vi "xiC - IMAQ - UpdateXiControl.vi"(6 "PRM_Attributes":T1={"Type"=enum."Int32", "Method"=enum."Get / Set", "Desc."="", "PRM"=enum."DEVICE_NAME"}, 8 "error in (no error)":errorcluster, 11 "Attributes In":T5) -> (0 "error out":errorcluster, 3 "Attributes Out":T5)   [LabVIEW 2015]
uses:
  xiCamLib/xiLIB/Typedefs/xiLIB - PRM_Function.ctl
  xiC - IMAQ - Attributes.ctl
  C:/GIT/Cameras3.x/Integrations/Labview/xiLib/xiLIB_32bit/xiLIB/xiCamLib/API/x86/xiApi.NET.dll
  xiLIB_32bit/xiLIB/xiCamLib/API/x86/xiApi.NET.dll
  xiCamLib/xiLIB/Typedefs/xiLIB - PRM_Type.ctl
  xiCamLib/xiLIB/Typedefs/xiLIB - PRM_Attribute.ctl
  xiC - IMAQ - TreeDisplayType.ctl
  xiCamLib/xiCam/PRM/PRM/PRM_v2.ctl
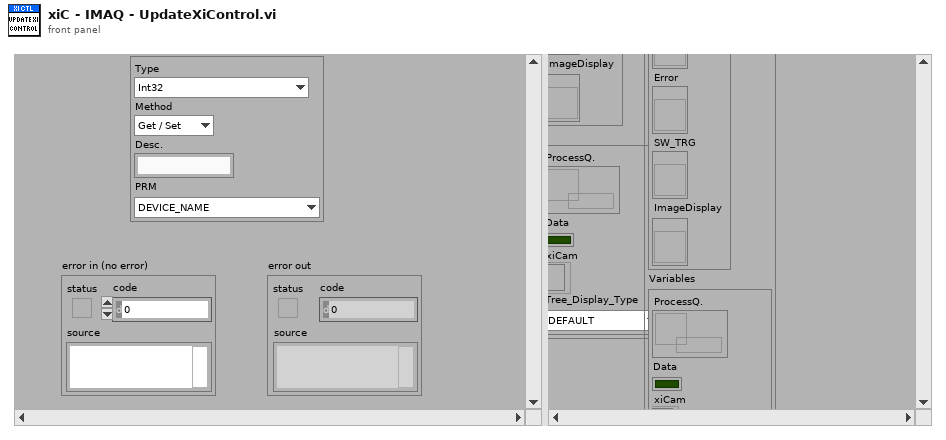
[diagram p1: front panel]
types:
  T1 = typedef "xiLIB - PRM_Attribute.ctl" = cluster{"Type":T2, "Method":T3, "Desc.":string, "PRM":T4}
  T2 = typedef "xiLIB - PRM_Type.ctl" = enum16{"Int32", "Float", "String", "DOWNSAMPLING_TYPE", "IMAGE_DATA_FORMAT", "BUFFER_POLICY", "TRG_SOURCE", "GPI", "GPO", "ACQ_TIMING_MODE", "BINNING_PATTERN", "BINNING_SELECTOR", "CMS_MODE", "COUNTER_SELECTOR", "DEBUG_LEVEL", "DECIMATION_PATTERN", "DECIMATION_SELECTOR", "GAIN_SELECTOR_TYPE", "LED_MODE", "LENS_FEATURE_SELECTOR", "LENS_MODE", "OUTPUT_DATA_PACKING_TYPE", "SENSOR_FEATURE_SELECTOR", "SHUTTER_TYPE", "TRG_SELECTOR", "TS_RST_MODE", "TS_RST_SOURCE"}
  T3 = typedef "xiLIB - PRM_Function.ctl" = enum16{"Get / Set", "Get", "Set"}
  T4 = typedef "PRM_v2.ctl" = enum16{"ACQ_BUFFER_SIZE", "ACQ_FRAME_BURST_COUNT", "ACQ_TIMING_MODE", "ACQ_TRANSPORT_BUFFER_SIZE", "AE_MAX_LIMIT", "AEAG", "AEAG_LEVEL", "API_VERSION", "AG_MAX_LIMIT", "APPLY_CMS", "AUTO_BANDWIDTH_CALCULATION", "AUTO_WB", "AVAILABLE_BANDWIDTH", "AVAILABLE_BANDWIDTH_MAX", "AVAILABLE_BANDWIDTH_MIN", "BPC", "BUFFER_POLICY", "BUFFERS_QUEUE_SIZE", "CC_MATRIX_00", "CC_MATRIX_01", "CC_MATRIX_02", "CC_MATRIX_03", "CC_MATRIX_10", "CC_MATRIX_11", "CC_MATRIX_12", "CC_MATRIX_13", "CC_MATRIX_20", "CC_MATRIX_21", "CC_MATRIX_22", "CC_MATRIX_23", "CC_MATRIX_30", "CC_MATRIX_31", "CC_MATRIX_32", "CC_MATRIX_33", "CHIP_TEMP", "CMS", "COLOR_FILTER_ARRAY", "COOLING", "DEBOUNCE_EN", "DEBOUNCE_POL", "DEBOUNCE_T0", "DEBOUNCE_T1", "DEBUG_LEVEL", "DEFAULT_CC_MATRIX", "DEVICE_INSTANCE_PATH", "DEVICE_MODEL_ID", "DEVICE_NAME", "DEVICE_SN", "DEVICE_TYPE", "DEVICE_USER_ID", "DOWNSAMPLING", "DOWNSAMPLING_MAX", "DOWNSAMPLING_MIN", "DOWNSAMPLING_TYPE", "DRV_VERSION", "EXP_PRIORITY", "EXPOSURE", "EXPOSURE_DIRECT_UPDATE", "EXPOSURE_MAX", "EXPOSURE_MIN", "FFS_FILE_NAME", "FPGA1_VERSION", "FRAMERATE", "FRAMERATE_MAX", "FRAMERATE_MIN", "FREE_FFS_SIZE", "GAIN", "GAIN_DIRECT_UPDATE", "GAIN_MAX", "GAIN_MIN", "GAMMAC", "GAMMAY", "GPI_LEVEL", "GPI_MODE", "GPI_SELECTOR", "GPI_SELECTOR_MAX", "GPI_SELECTOR_MIN", "GPO_MODE", "GPO_SELECTOR", "GPO_SELECTOR_MAX", "GPO_SELECTOR_MIN", "HDR", "HDR_T1", "HDR_T2", "HEIGHT", "HEIGHT_MAX", "HEIGHT_MIN", "HOUSE_TEMP", "IMAGE_DATA_FORMAT", "IMAGE_IS_COLOR", "INPUT_CMS_PROFILE", "IS_COOLED", "IS_DEVICE_EXIST", "KNEEPOINT1", "KNEEPOINT2", "LED_MODE", "LED_SELECTOR", "LED_SELECTOR_MAX", "LED_SELECTOR_MIN", "LIMIT_BANDWIDTH", "LIMIT_BANDWIDTH_MAX", "LIMIT_BANDWIDTH_MIN", "LUT_EN", "LUT_INDEX", "LUT_INDEX_MAX", "LUT_INDEX_MIN", "LUT_VALUE", "LUT_VALUE_MAX", "LUT_VALUE_MIN", "MANUAL_WB", "MCU1_VERSION", "MCU2_VERSION", "OFFSET_X", "OFFSET_X_MAX", "OFFSET_X_MIN", "OFFSET_Y", "OFFSET_Y_MAX", "OFFSET_Y_MIN", "OUTPUT_CMS_PROFILE", "OUTPUT_DATA_BIT_DEPTH", "OUTPUT_DATA_PACKING", "READ_FILE_FFS", "RECENT_FRAME", "SENSOR_DATA_BIT_DEPTH", "SENSOR_MODE", "SENSOR_TAPS", "SHARPNESS", "SHUTTER_TYPE", "TARGET_TEMP", "TRG_DELAY", "TRG_SELECTOR", "TRG_SOFTWARE", "TRG_SOURCE", "USED_FFS_SIZE", "WB_KB", "WB_KG", "WB_KR", "WIDTH", "WIDTH_MAX", "WIDTH_MIN", "WRITE_FILE_FFS", "ACQ_BUFFER_SIZE_UNIT", "ACQ_TRANSPORT_BUFFER_COMMIT", "AEAG_ROI_HEIGHT", "AEAG_ROI_OFFSET_X", "AEAG_ROU_OFFSET_Y", "AEAG_ROI_WIDTH", "API_CONTEXT_LIST", "BINNING_HORIZONTAL", "BINNING_SELECTOR", "BINNING_VERTICAL", "COLUMN_FPN_CORRECTION", "COUNTER_SELECTOR", "COUNTER_VALUE", "DECIMATION_HORIZONTAL", "DECIMATION_SELECTOR", "DECIMATION_VERTICAL", "DEVICE_ID", "DEVICE_LOCATION_PATH", "DEVICE_MANIFEST", "DEVICE_RESET", "DEVICE_SENS_SN", "EXPOSURE_BURST_COUNT", "FFS_ACCESS_KEY", "GAIN_SELECTOR", "HW_REVISION", "IMAGE_BLACK_LEVEL", "IMAGE_DATA_BIT_DEPTH", "IMAGE_DATA_FORMAT_RGB32_ALPHA", "IMAGE_PAYLOAD_SIZE", "LENS_APERTURE_VALUE", "LENS_FEATURE", "LENS_FEATURE_SELECTOR", "LENS_FOCAL_LENGTH", "LENS_FOCUS_DISTANCE", "LENS_FOCUS_MOVE", "LENS_FOCUS_MOVEMENT_VALUE", "LENS_MODE", "OUTPUT_DATA_PACKING_TYPE", "SENSOR_CLOCK_FREQ_HZ", "SENSOR_CLOCK_FREQ_INDEX", "SENSOR_FEATURE_SELECTOR", "SENSOR_FEATURE_VALUE", "SENSOR_OUTPUT_CHANNEL_COUNT", "TRANSPORT_PIXEL_FORMAT", "TS_RST_MODE", "TS_RST_SOURCE"}
  T5 = typedef "xiC - IMAQ - Attributes.ctl" = cluster{"Controls":cluster{"VI Ref.":refnum<vi>, "Tree":refnum<vi>, "Info":refnum<vi>, "PRMName":refnum<vi>, "xiControl":refnum<vi>, "Error":refnum<vi>, "SW_TRG":refnum<vi>, "ImageDisplay":refnum<vi>}, "Variables":cluster{"ProcessQ.":refnum<queue>, "Data":bool, "xiCam":refnum<k24>, "Tree_Display_Type":T6}}
  T6 = typedef "xiC - IMAQ - TreeDisplayType.ctl" = enum16{"DEFAULT", "HIDE_MAX_MIN"}
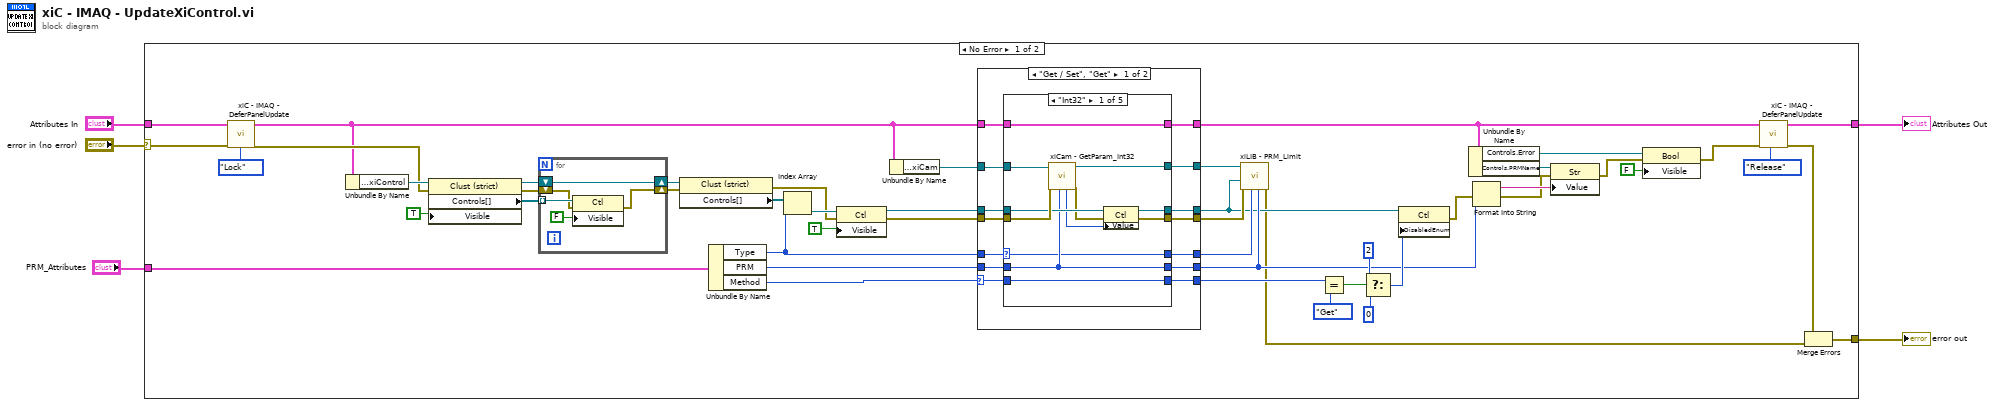
[diagram p0: block diagram]
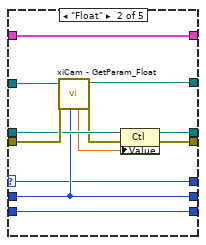
[diagram p2: hidden frame]
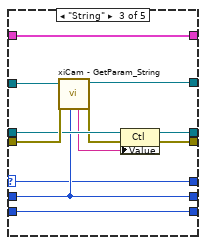
[diagram p3: hidden frame]
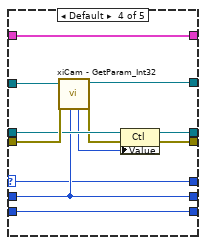
[diagram p4: hidden frame]
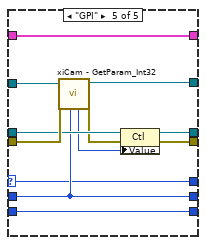
[diagram p5: hidden frame]
diagram:
  n1 = case shown="No Error" "error in (no error)" {
    selector: "error in (no error)" -> [w50 w141]
    tunnel: [w6 w141] -> w4
    tunnel: "Attributes In" -> [w53 w140]
    tunnel: [w49 w140] -> w2
    tunnel: "PRM_Attributes" -> [w47 _]
    frame No Error {
      n2 = call "xiC - IMAQ - DeferPanelUpdate.vi"("Operand"=enum16{"Lock", "Release"}."Lock", "error in (no error)"=w50, "Attributes"=w53) -> ("error out"=w44:errorcluster, "Attributes"=w33:T5)  [unwired: 7 in]
      n3 = Unbundle By Name(w33) -> ("Controls.xiControl"=w46:refnum<vi>)
      n4 = property class="Clust (strict)"(reference=w46, error in=w44, "Visible"=TRUE) -> (reference out=w42:refnum<vi>, error out=w43:errorcluster, "Controls[]"=w45:refnum<vi>[])
      n5 = for {
        tunnel: w45 -> [w139] mode=indexing
        shift-right: [w136] -> w40
        shift-left: w43 -> [w137]
        shift-right: [w135] -> w41
        shift-left: w42 -> [w135]
        n6 = property class="Ctl"(reference=w139, error in=w137, "Visible"=FALSE) -> (error out=w136:errorcluster)  [unwired: 1 out]
      }
      n7 = property class="Clust (strict)"(reference=w41, error in=w40) -> (error out=w37:errorcluster, "Controls[]"=w39:refnum<vi>[])  [unwired: 1 out]
      n8 = Unbundle By Name(w47) -> ("Type"=w30:T2, "PRM"=w31:T4, "Method"=w21:T3)
      n9 = Index Array(array=w39, index=w30) -> (element=w38:refnum<vi>)
      n10 = property class="Ctl"(reference=w38, error in=w37, "Visible"=TRUE) -> (reference out=w35:refnum<vi>, error out=w34:errorcluster)
      n11 = Unbundle By Name(w33) -> ("Variables.xiCam"=w32:refnum<k24>)
      n12 = case shown="\"Get / Set\", \"Get\"" w21 {
        selector: w21 -> [w59 w132]
        tunnel: w35 -> [w63 w131]
        tunnel: w34 -> [w65 w133]
        tunnel: w33 -> [w61 w134]
        tunnel: w32 -> [w66 w128]
        tunnel: w31 -> [w64 w130]
        tunnel: w30 -> [w67 w129]
        tunnel: [w62 w133] -> w12
        tunnel: [w60 w134] -> w22
        tunnel: [w58 w132] -> w29
        tunnel: [w57 w131] -> w9
        tunnel: [w56 w130] -> w10
        tunnel: [w55 w129] -> w11
        tunnel: [w54 w128] -> w13
        frame "Get / Set", "Get" {
          n13 = case shown="\"Int32\"" w67 {
            selector: w67 -> [w69 w81 w93 w105 w117]
            tunnel: w66 -> [w79 w91 w103 w115 w127]
            tunnel: w65 -> [w78 w90 w102 w114 w126]
            tunnel: w64 -> [w70 w82 w94 w106 w118]
            tunnel: w63 -> [w77 w89 w101 w113 w125]
            tunnel: [w74 w86 w98 w110 w122] -> w62
            tunnel: w61 -> [w73 w85 w97 w109 w121]
            tunnel: [w73 w85 w97 w109 w121] -> w60
            tunnel: w59 -> [w72 w84 w96 w108 w120]
            tunnel: [w72 w84 w96 w108 w120] -> w58
            tunnel: [w71 w83 w95 w107 w119] -> w57
            tunnel: [w70 w82 w94 w106 w118] -> w56
            tunnel: [w69 w81 w93 w105 w117] -> w55
            tunnel: [w68 w80 w92 w104 w116] -> w54
            frame "Int32" {
              n14 = call "xiCam - GetParam_Int32.vi"("PRM"=w70, "error in (no error)"=w78, "xiCam In"=w79) -> ("error out"=w76:errorcluster, "xiCam Out"=w68:refnum<k24>, "Int32_Value"=w75:i32)  [unwired: 6 in]
              n15 = property class="Ctl"(reference=w77, error in=w76, "Value"=w75) -> (reference out=w71:refnum<vi>, error out=w74:errorcluster)
            }
            frame "Float" {
              n16 = call "xiCam - GetParam_Float.vi"("PRM"=w82, "error in (no error)"=w90, "xiCam In"=w91) -> ("error out"=w88:errorcluster, "xiCam Out"=w80:refnum<k24>, "Float_Value"=w87:sgl)  [unwired: 6 in]
              n17 = property class="Ctl"(reference=w89, error in=w88, "Value"=w87) -> (reference out=w83:refnum<vi>, error out=w86:errorcluster)
            }
            frame "String" {
              n18 = call "xiCam - GetParam_String.vi"("PRM"=w94, "error in (no error)"=w102, "xiCam In"=w103) -> ("error out"=w100:errorcluster, "xiCam Out"=w92:refnum<k24>, "String_Value"=w99:string)  [unwired: 6 in]
              n19 = property class="Ctl"(reference=w101, error in=w100, "Value"=w99) -> (reference out=w95:refnum<vi>, error out=w98:errorcluster)
            }
            frame Default {
              n20 = call "xiCam - GetParam_Int32.vi"("PRM"=w106, "error in (no error)"=w114, "xiCam In"=w115) -> ("error out"=w112:errorcluster, "xiCam Out"=w104:refnum<k24>, "Int32_Value"=w111:i32)  [unwired: 6 in]
              n21 = property class="Ctl"(reference=w113, error in=w112, "Value"=w111) -> (reference out=w107:refnum<vi>, error out=w110:errorcluster)
            }
            frame "GPI" {
              n22 = call "xiCam - GetParam_Int32.vi"("PRM"=w118, "error in (no error)"=w126, "xiCam In"=w127) -> ("error out"=w124:errorcluster, "xiCam Out"=w116:refnum<k24>, "Int32_Value"=w123:i32)  [unwired: 6 in]
              n23 = property class="Ctl"(reference=w125, error in=w124, "Value"=w123) -> (reference out=w119:refnum<vi>, error out=w122:errorcluster)
            }
          }
        }
        frame "Set" {
        }
      }
      n24 = call "xiLIB - PRM_Limit.vi"("PRM"=w10, "Type"=w11, "error in (no error)"=w12, "Ctl Refnum"=w9, "xiCam In"=w13) -> ("error out"=w7:errorcluster)  [unwired: 5 in, 1 out]
      n25 = Equal?(x=w29, y=xiLIB_-_PRM_Function."Get") -> (x = y?=w27:bool)
      n26 = Select(t=2, s=w27, f=0) -> (s? t:f=w25:i32)
      n27 = property class="Ctl"(reference=w9, "DisabledEnum"=w25) -> (error out=w23:errorcluster)  [unwired: 1 in, 1 out]
      n28 = Unbundle By Name(w22) -> ("Controls.Error"=w16:refnum<vi>, "Controls.PRMName"=w20:refnum<vi>)
      n29 = Format Into String(error in=w23, w10) -> (resulting string=w48:string, error out=w19:errorcluster)  [unwired: 2 in]
      n30 = property class="Str"(reference=w20, error in=w19, "Value"=w48) -> (error out=w15:errorcluster)  [unwired: 1 out]
      n31 = property class="Bool"(reference=w16, error in=w15, "Visible"=FALSE) -> (error out=w14:errorcluster)  [unwired: 1 out]
      n32 = call "xiC - IMAQ - DeferPanelUpdate.vi"("Operand"=enum16{"Lock", "Release"}."Release", "error in (no error)"=w14, "Attributes"=w22) -> ("error out"=w8:errorcluster, "Attributes"=w49:T5)  [unwired: 7 in]
      n33 = Merge Errors(w8, w7) -> (w6:errorcluster)
    }
    frame Error {
    }
  }
  "error out" <- w4
  "Attributes Out" <- w2
